vi "Play Channel.vi"(6 "Ticks":i32, 8 "error in":errorcluster, 9 "Loops":i32, 10 "Chunk Pointer":u32 format="%.0x", 11 "Channel":i32) -> (0 "error out":errorcluster, 3 "Channel":i32)   [LabVIEW 2015, in "LibSDL2_Mixer.lvlib"]
uses:
  LibSDL2_Mixer.lvlib
  LibSDL2 Wrapper/DLL/SDL2_mixer.dll
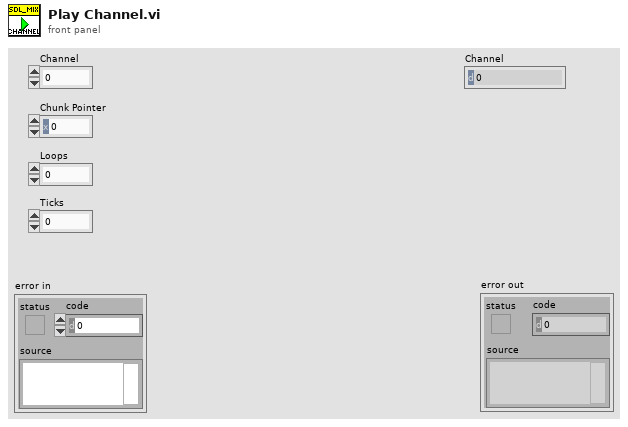
[diagram p1: front panel]
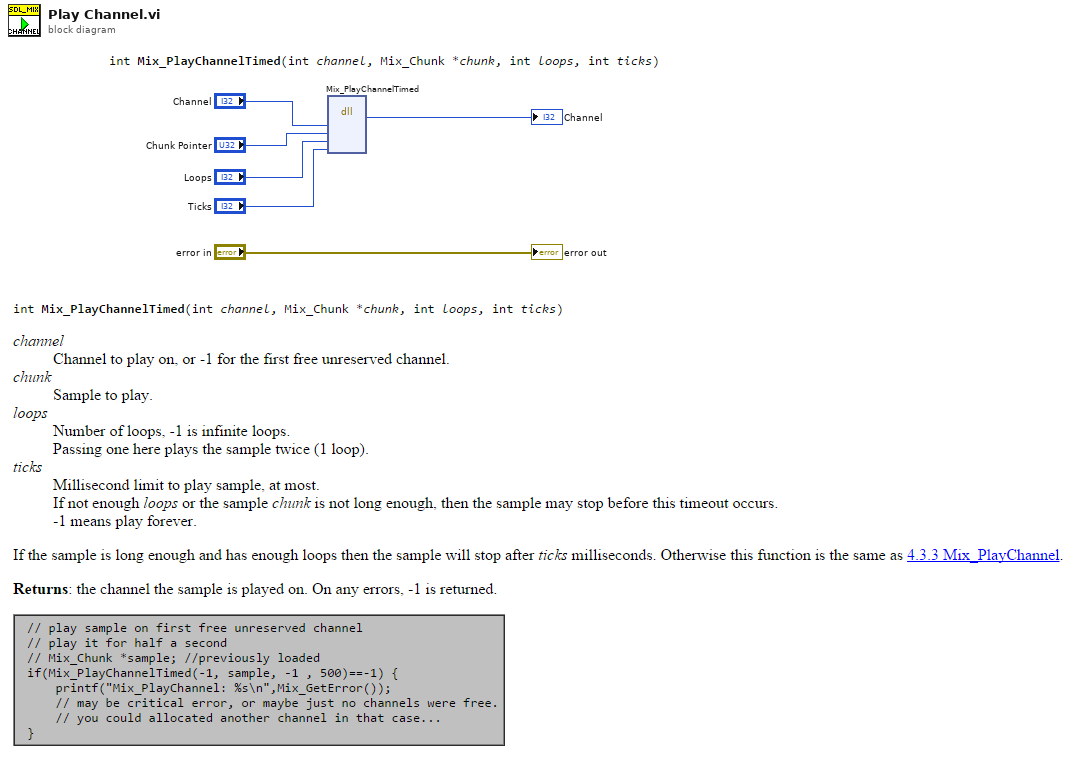
[diagram p0: block diagram]
diagram:
  n1 = dll-call lib="C:/dev/PGS/LabSDL2/Source/Libraries/LibSDL2 Wrapper/DLL/SDL2_mixer.dll" fn="Mix_PlayChannelTimed"("channel"="Channel", "chunkptr"="Chunk Pointer", "loops"="Loops", "ticks"="Ticks") -> ("return type"=→"Channel":i32)  [unwired: 7 in, 2 out]
  "error out" <- "error in"
